vi "rt nominal connect.vi"(8 "error in":errorcluster, 11 "stream configuration":T5={"stream name"="", "Base URL"="https://api.gov.nominal.io/api/", "api key"="", "identifier selection"=enum."Asset Identifier and Dataset Name", "asset ID"="", "dataset name"="", "dataset ID"="", "associated channels"=[], "fallback avro path"=path "", "time source"=enum."to timestamp", "buffer size"=0}) -> (0 "error out":errorcluster, 2 "channel buffer":T1, 3 "nominal state":T3)   [LabVIEW 2026, in "Nominal Core Streaming Engine.lvlib"]
uses:
  Nominal Core Streaming Engine.lvlib
  Shared/compiled stream data.ctl
  Shared/stream configuration mode.ctl
  Shared/time convert type.ctl
  nominal runtime state.ctl
  rt full channel buffer.ctl
  rt per channel buffer.ctl
  <vilib>/Utility/sysdir.llb/System Directory Type.ctl
  Shared/Nominal Core Streaming Shared.lvlib
  lib_nominal-streaming-lv_64.dll
  libnominalClient_64.dll
panel:
  out "out_stream_handle":u64
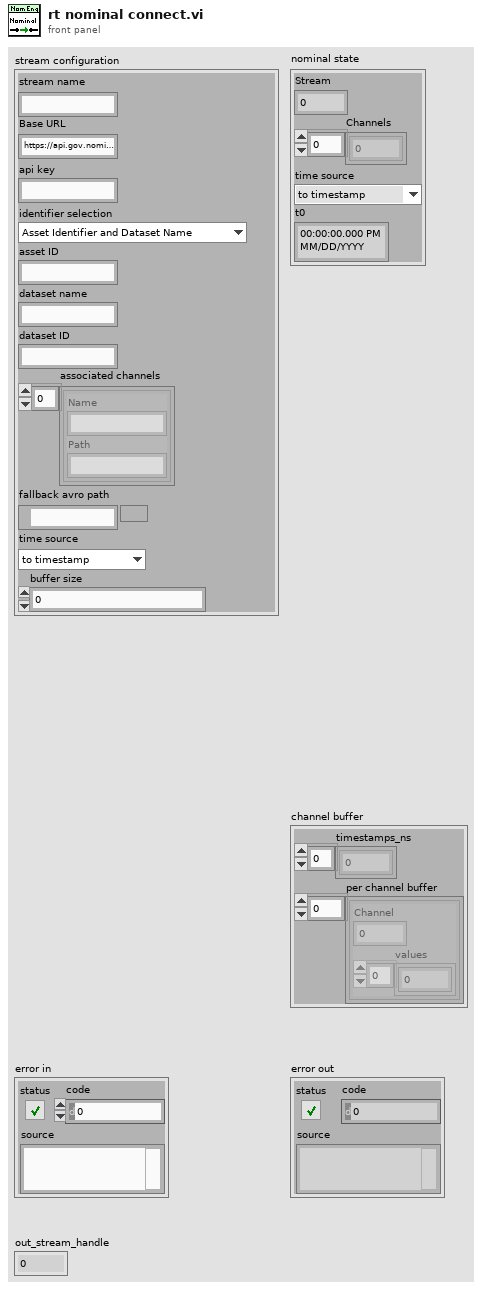
[diagram p1: front panel]
types:
  T1 = typedef "Nominal Core Streaming Engine.lvlib/rt full channel buffer.ctl" = cluster{"timestamps_ns":i64[], "per channel buffer":T2[]}
  T2 = typedef "Nominal Core Streaming Engine.lvlib/rt per channel buffer.ctl" = cluster{"Channel":u64, "values":dbl[]}
  T3 = typedef "Nominal Core Streaming Engine.lvlib/nominal runtime state.ctl" = cluster{"Stream":u64, "Channels":u64[], "time source":T4, "t0":timestamp}
  T4 = typedef "Nominal Core Streaming Shared.lvlib/time convert type.ctl" = enum16{"to timestamp", "relative seconds"}
  T5 = typedef "Nominal Core Streaming Shared.lvlib/compiled stream data.ctl" = cluster{"stream name":string, "Base URL":string, "api key":string, "identifier selection":T6, "asset ID":string, "dataset name":string, "dataset ID":string, "associated channels":cluster{"Name":string, "Path":string}[], "fallback avro path":path, "time source":T4, "buffer size":u32}
  T6 = typedef "Nominal Core Streaming Shared.lvlib/stream configuration mode.ctl" = enum16{"Asset Identifier and Dataset Name", "Dataset Identifier"}
  T7 = typedef "System Directory Type.ctl" = i32
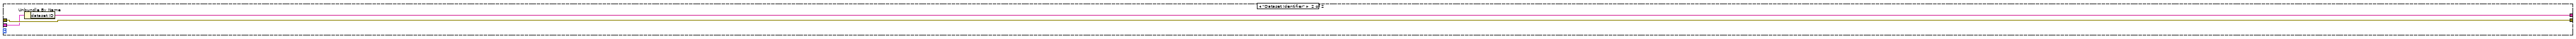
[diagram p4: hidden frame]
diagram:
  n1 = Unbundle By Name("stream configuration") -> ("associated channels"=w15:cluster{"Name":string, "Path":string}[])
  n2 = Unbundle By Name("stream configuration") -> ("identifier selection"=w21:T6)
  n3 = Unbundle By Name("stream configuration") -> ("fallback avro path"=w19:path)
  n4 = Unbundle By Name("stream configuration") -> ("time source"=w9:T4)
  n5 = Unbundle By Name("stream configuration") -> ("buffer size"=w4:u32)
  n6 = case shown="\"Asset Identifier and Dataset Name\"" w21 {
    tunnel: "error in" -> [w29 w164]
    tunnel: [w25 w164] -> w2
    tunnel: "stream configuration" -> [w23 w163]
    tunnel: [w28 w162] -> w1
    frame "Asset Identifier and Dataset Name" {
      n7 = flat-sequence {
        tunnel: [w53] -> w36
        tunnel: [w52] -> w35
        tunnel: w29 -> [w51]
        tunnel: [w49] -> w26
        tunnel: [w48] -> w24
        tunnel: w23 -> [w38]
        frame #0 {
          n8 = Unbundle By Name(w38) -> ("api key"=w39:string, "Base URL"=w40:string)
          n9 = Unbundle By Name(w38) -> ("asset ID"=w37:string)
          n10 = dll-call lib="C:/sw/ni-veristand-custom-device-nominal-core/source/libnominalClient_*.*" fn="nominal_client_new"(error in=w51, "token"=w39, "workspace_rid"="", "base_url"=w40) -> (error out=w42:errorcluster, "return type"=w41:i32, "out_client"=w48:i32)  [unwired: 6 in, 1 out]
          n11 = call "extracted dll error handler.vi"("error in (no error)"=w42, "error code"=w41) -> ("error out"=w50:errorcluster)  [unwired: 9 in]
          n12 = dll-call lib="C:/sw/ni-veristand-custom-device-nominal-core/source/libnominalClient_*.*" fn="nominal_asset_get"(error in=w50, "client"=w48, "rid"=w37) -> (error out=w45:errorcluster, "return type"=w44:i32, "out_asset"=w49:i32)  [unwired: 5 in, 1 out]
          n13 = call "extracted dll error handler.vi"("error in (no error)"=w45, "error code"=w44) -> ("error out"=w54:errorcluster)  [unwired: 9 in]
          n14 = dll-call lib="C:/sw/ni-veristand-custom-device-nominal-core/source/libnominalClient_*.*" fn="nominal_asset_data_source_count"(error in=w54, "asset"=w49) -> (error out=w47:errorcluster, "return type"=w46:i32, "out_count"=w52:u32)  [unwired: 4 in, 1 out]
          n15 = call "extracted dll error handler.vi"("error in (no error)"=w47, "error code"=w46) -> ("error out"=w53:errorcluster)  [unwired: 9 in]
        }
      }
      n16 = for {
        N: w35 -> [_]
        shift-right: [w93] -> w31
        shift-left: w36 -> [w95]
        tunnel: w26 -> [w91]
        tunnel: [w89] -> w30
        tunnel: [w88] -> w34
        tunnel: w24 -> [w87]
        tunnel: w23 -> [w86]
        i -> [w90]
        stop <- w88 stop-if-true
        n17 = flat-sequence {
          tunnel: w95 -> [w102]
          tunnel: [w101] -> w94
          tunnel: [w100] -> w92
          tunnel: w91 -> [w99]
          tunnel: w90 -> [w98]
          frame #0 {
            # "NominalDataSourceType_Dataset = 0,\n  NominalDataSourceType_Video = 1,\n  NominalDataSourceType_Connection = 2,"
            n18 = dll-call lib="C:/sw/ni-veristand-custom-device-nominal-core/source/libnominalClient_*.*" fn="nominal_asset_data_source_type_at"(error in=w102, "asset"=w99, "index"=w98) -> (error out=w97:errorcluster, "return type"=w96:i32, "out_type"=w101:i32)  [unwired: 5 in, 1 out]
            n19 = call "extracted dll error handler.vi"("error in (no error)"=w97, "error code"=w96) -> ("error out"=w100:errorcluster)  [unwired: 9 in]
          }
        }
        n20 = case shown="0" w94 {
          tunnel: [w105 w161] -> w93
          tunnel: w92 -> [w119 w161]
          tunnel: w91 -> [w118 _]
          tunnel: w90 -> [w114 _]
          tunnel: [w110 _] -> w89
          tunnel: [w107 _] -> w88
          tunnel: w87 -> [w111 _]
          tunnel: w86 -> [w104 _]
          frame 0 {
            # "I personally find scope name vs dataset name to be extremely confusing, so I'm checking both"
            n21 = stacked-sequence {
              tunnel: [w132] -> w117
              tunnel: [w128] -> w116
              tunnel: [w125] -> _
              tunnel: [w129] -> _
              tunnel: w119 -> [w130]
              tunnel: w114 -> [w127]
              tunnel: w118 -> [w126]
              frame #0 {
                n22 = call "extracted create string buffer.vi"("Buffer Size (1024)"=2048 ("dimension size")) -> ("dub Buffer Size"=w123:i32, "String Buffer"=w122:string)  [unwired: 8 in, 1 out]
                n23 = dll-call lib="C:/sw/ni-veristand-custom-device-nominal-core/source/libnominalClient_*.*" fn="nominal_asset_data_source_name_at"(error in=w130, "asset"=w126, "index"=w127, "buf"=w122, "cap"=w123) -> (error out=w131:errorcluster, "return type"=w125:i32, "buf"=w128:string, "out_needed"=w129:u32)  [unwired: 6 in, 1 out]
                n24 = call "extracted dll error handler.vi"("error in (no error)"=w131, "error code"=w125) -> ("error out"=w132:errorcluster)  [unwired: 9 in]
              }
            }
            n25 = Unbundle By Name(w104) -> ("dataset name"=w103:string)
            n26 = Equal?(x=w103, y=w116) -> (x = y?=w115:bool)
            n27 = stacked-sequence {
              tunnel: [w143] -> w112
              tunnel: [w139] -> w110
              tunnel: [w136] -> _
              tunnel: [w140] -> _
              tunnel: w117 -> [w141]
              tunnel: w114 -> [w138]
              tunnel: w118 -> [w137]
              frame #0 {
                n28 = call "extracted create string buffer.vi"("Buffer Size (1024)"=2048 ("dimension size")) -> ("dub Buffer Size"=w134:i32, "String Buffer"=w133:string)  [unwired: 8 in, 1 out]
                n29 = dll-call lib="C:/sw/ni-veristand-custom-device-nominal-core/source/libnominalClient_*.*" fn="nominal_asset_data_source_rid_at"(error in=w141, "asset"=w137, "index"=w138, "buf"=w133, "cap"=w134) -> (error out=w142:errorcluster, "return type"=w136:i32, "buf"=w139:string, "out_needed"=w140:u32)  [unwired: 6 in, 1 out]
                n30 = call "extracted dll error handler.vi"("error in (no error)"=w142, "error code"=w136) -> ("error out"=w143:errorcluster)  [unwired: 9 in]
              }
            }
            n31 = stacked-sequence {
              tunnel: [w160] -> w109
              tunnel: [w157] -> w113
              tunnel: [w154] -> _
              tunnel: w112 -> [w158]
              tunnel: w110 -> [w156]
              tunnel: w111 -> [w155]
              frame #0 {
                n32 = dll-call lib="C:/sw/ni-veristand-custom-device-nominal-core/source/libnominalClient_*.*" fn="nominal_dataset_get"(error in=w158, "client"=w155, "rid"=w156) -> (error out=w159:errorcluster, "return type"=w154:i32, "out_dataset"=w157:i32)  [unwired: 5 in, 1 out]
                n33 = call "extracted dll error handler.vi"("error in (no error)"=w159, "error code"=w154) -> ("error out"=w160:errorcluster)  [unwired: 9 in]
              }
            }
            n34 = stacked-sequence {
              tunnel: [w153] -> w105
              tunnel: [w149] -> w108
              tunnel: [w147] -> _
              tunnel: [w150] -> _
              tunnel: w109 -> [w151]
              tunnel: w113 -> [w148]
              frame #0 {
                n35 = call "extracted create string buffer.vi"("Buffer Size (1024)"=2048 ("dimension size")) -> ("dub Buffer Size"=w145:i32, "String Buffer"=w144:string)  [unwired: 8 in, 1 out]
                n36 = dll-call lib="C:/sw/ni-veristand-custom-device-nominal-core/source/libnominalClient_*.*" fn="nominal_dataset_name"(error in=w151, "dataset"=w148, "buf"=w144, "cap"=w145) -> (error out=w152:errorcluster, "return type"=w147:i32, "buf"=w149:string, "out_needed"=w150:u32)  [unwired: 5 in, 1 out]
                n37 = call "extracted dll error handler.vi"("error in (no error)"=w152, "error code"=w147) -> ("error out"=w153:errorcluster)  [unwired: 9 in]
              }
            }
            n38 = Equal?(x=w103, y=w108) -> (x = y?=w106:bool)
            n39 = flat-sequence {
              tunnel: w113 -> [w121]
              tunnel: w105 -> [_]
              tunnel: [w120] -> _
              frame #0 {
                n40 = dll-call lib="C:/sw/ni-veristand-custom-device-nominal-core/source/libnominalClient_*.*" fn="nominal_dataset_free"("dataset"=w121) -> (error out=w120:errorcluster)  [unwired: 5 in, 1 out]
              }
            }
            n41 = Or(x=w106, y=w115) -> (x .or. y?=w107:bool)
          }
          frame Default {
          }
        }
      }
      n42 = Empty String/Path?(string/path=w30) -> (empty?=w33:bool)
      n43 = Compound Arithmetic op=AND(invert w33, w34) -> (w32:bool)
      n44 = case shown="False" w32 {
        tunnel: w31 -> [w81 w85]
        tunnel: w24 -> [w71 _]
        tunnel: w30 -> [_ w84]
        tunnel: [w73 w85] -> w25
        tunnel: [w66 w84] -> w28
        tunnel: w23 -> [w69 _]
        frame False {
          # "not found on asset, create and attach"
          n45 = Unbundle By Name(w69) -> ("dataset name"=w67:string, "stream name"=w68:string)
          n46 = dll-call lib="C:/sw/ni-veristand-custom-device-nominal-core/source/libnominalClient_*.*" fn="nominal_dataset_create"(error in=w81, "client"=w71, "name"=w67, "description"=w68) -> (error out=w65:errorcluster, "return type"=w64:i32, "out_dataset"=w72:i32)  [unwired: 6 in, 1 out]
          n47 = Unbundle By Name(w69) -> ("asset ID"=w70:string, "dataset name"=w59:string)
          n48 = call "extracted dll error handler.vi"("error in (no error)"=w65, "error code"=w64) -> ("error out"=w75:errorcluster)  [unwired: 9 in]
          n49 = call "extracted create string buffer.vi"("error in"=w75, "Buffer Size (1024)"=2048) -> ("error out"=w79:errorcluster, "dub Buffer Size"=w77:i32, "String Buffer"=w78:string)  [unwired: 7 in]
          n50 = dll-call lib="C:/sw/ni-veristand-custom-device-nominal-core/source/libnominalClient_*.*" fn="nominal_dataset_rid"(error in=w79, "dataset"=w72, "buf"=w78, "cap"=w77, "out_needed"=u32 0) -> (error out=w61:errorcluster, "return type"=w60:i32, "buf"=w66:string)  [unwired: 5 in, 1 out]
          n51 = call "extracted dll error handler.vi"("error in (no error)"=w61, "error code"=w60) -> ("error out"=w74:errorcluster)  [unwired: 9 in]
          n52 = dll-call lib="C:/sw/ni-veristand-custom-device-nominal-core/source/libnominalClient_*.*" fn="nominal_asset_add_dataset"(error in=w74, "client"=w71, "rid"=w70, "scope_name"=w59, "dataset_rid"=w66) -> (error out=w63:errorcluster, "return type"=w62:i32, "out_asset"=w80:i32)  [unwired: 7 in, 1 out]
          n53 = flat-sequence {
            tunnel: w80 -> [w82]
            tunnel: w72 -> [w83]
            frame #0 {
              # "int32_t nominal_asset_free(int32_t asset);"
              n54 = dll-call lib="C:/sw/ni-veristand-custom-device-nominal-core/source/libnominalClient_*.*" fn="nominal_asset_free"("asset"=w82) -> ()  [unwired: 5 in, 2 out]
            }
            frame #1 {
              # "int32_t nominal_dataset_free(int32_t dataset);"
              n55 = dll-call lib="C:/sw/ni-veristand-custom-device-nominal-core/source/libnominalClient_*.*" fn="nominal_dataset_free"("dataset"=w83) -> ()  [unwired: 5 in, 2 out]
            }
          }
          n56 = call "extracted dll error handler.vi"("error in (no error)"=w63, "error code"=w62) -> ("error out"=w73:errorcluster)  [unwired: 9 in]
        }
        frame True {
          # "exists and is part of asset"
        }
      }
      n57 = flat-sequence {
        tunnel: w24 -> [w56]
        tunnel: [w56] -> w27
        tunnel: w26 -> [w55]
        tunnel: w25 -> [_]
        tunnel: w27 -> [w57]
        frame #0 {
          # "int32_t nominal_asset_free(int32_t asset);"
          n58 = dll-call lib="C:/sw/ni-veristand-custom-device-nominal-core/source/libnominalClient_*.*" fn="nominal_asset_free"("asset"=w55) -> ()  [unwired: 5 in, 2 out]
        }
        frame #1 {
          # "int32_t nominal_client_free(int32_t client);"
          n59 = dll-call lib="C:/sw/ni-veristand-custom-device-nominal-core/source/libnominalClient_*.*" fn="nominal_client_free"("client"=w57) -> ()  [unwired: 5 in, 2 out]
        }
      }
    }
    frame "Dataset Identifier" {
      n60 = Unbundle By Name(w163) -> ("dataset ID"=w162:string)
    }
  }
  n61 = call "reprocess channel names for duplicates.vi"("channels in"=w15) -> ("processed channels"=w14:cluster{"Name":string, "Path":string}[])  [unwired: 10 in]
  n62 = stacked-sequence {
    tunnel: [w177] -> w20
    tunnel: w19 -> [w188]
    tunnel: w2 -> [w191]
    tunnel: [w176] -> w7
    tunnel: "stream configuration" -> [w174]
    tunnel: w1 -> [w165]
    frame #0 {
      w183 = T7 2 items=["User Home"=0, "User Desktop"=1, "User Documents"=2, "User Application Data"=3, "User Preferences"=4, "User Temporary"=5, "Public Documents"=6, "Public Application Data"=7, "Public Preferences"=8, "Public Cache"=13, "System Core Libraries"=9, "System Installed Libraries"=10, "Application Files"=11, "Boot Volume Root"=12] ("system directory type")
      # "streaming setup"
      n63 = Unbundle By Name(w174) -> ("api key"=w175:string)
      n64 = call <vilib>:"Get System Directory.vi"("system directory type"=w183) -> ("system directory"=w182:path)  [unwired: 10 in]
      n65 = Get Date/Time In Seconds() -> (seconds since 1Jan1904=w180:timestamp)
      n66 = Build Path(base path=w182, name or relative path=path "nominal_fallback_files") -> (appended path=w184:path)
      n67 = Format Into String(format string="%<%Y-%m-%d_%H-%M_fallback-file.avro>T", error in=w191, w180) -> (resulting string=w181:string, error out=w186:errorcluster)  [unwired: 1 in]
      n68 = call <vilib>:"Is Path and Not Empty.vi"("path"=w188) -> ("Is Path and Not Empty?"=w187:bool)  [unwired: 4 in]
      n69 = call <vilib>:"Create Directory Recursive.vi"("error in (no error)"=w186, "directory"=w184) -> ("directory copy"=w185:path)  [unwired: 3 in, 2 out]
      n70 = Build Path(base path=w185, name or relative path=w181) -> (appended path=w189:path)
      n71 = Select(t=w188, s=w187, f=w189) -> (s? t:f=w190:path)
      n72 = Path To String(path=w190) -> (string=w172:string)
      n73 = dll-call lib="C:/sw/ni-veristand-custom-device-nominal-core/source/lib_nominal-streaming-lv_*.*" fn="nominal_init"(error in=w191, "token"=w175, "dataset_rid"=w165, "fallback_file_path"=w172, "out_stream_handle"=u64 0) -> (error out=w173:errorcluster, "out_stream_handle"=w176:u64)  [unwired: 6 in, 1 out]
      n74 = call "extracted create string buffer.vi"() -> ("dub Buffer Size"=w166:i32, "String Buffer"=w167:string)  [unwired: 9 in, 1 out]
      n75 = dll-call lib="C:/sw/ni-veristand-custom-device-nominal-core/source/lib_nominal-streaming-lv_*.*" fn="nominal_get_last_error"(error in=w173, "buffer"=w167, "buffer_size"=w166) -> (error out=w168:errorcluster, "return type"=w170:i32, "buffer"=w169:string)  [unwired: 3 in, 1 out]
      n76 = case shown="Default" w170 {
        tunnel: w168 -> [w192 w197]
        tunnel: [w192 w196] -> w177
        tunnel: w169 -> [_ w195]
        frame -1 {
        }
        frame Default {
          n77 = call <vilib>:"Error Cluster From Error Code.vi"("show call chain? (False)"=TRUE, "error in (no error)"=w197, "error message (\"\")"=w195, "error code (0)"=5001) -> ("error out"=w196:errorcluster)  [unwired: 5 in]
        }
      }
    }
  }
  "out_stream_handle" <- w7
  n78 = for {
    shift-right: [w210] -> w16
    shift-left: w20 -> [w211]
    tunnel: w14 -> [w208] mode=indexing
    tunnel: [w203] -> w11 mode=indexing
    tunnel: w4 -> [w200]
    tunnel: [w198] -> w8 mode=indexing
    tunnel: w7 -> [w199]
    n79 = Unbundle(w208) -> ("Name"=w205:string, "Path"=w207:string)
    n80 = node("nivs_path" ("key"), w207) -> (w209:map{string, string})
    n81 = stacked-sequence {
      tunnel: [w225] -> w210
      tunnel: w211 -> [w219]
      tunnel: w209 -> [w221]
      tunnel: w205 -> [w227]
      tunnel: [w218] -> w198
      tunnel: w199 -> [w217]
      frame #0 {
        n82 = for {
          tunnel: w221 -> [w238] mode=indexing
          tunnel: [w234] -> w222 mode=indexing
          n83 = Unbundle By Name(w238) -> ("key"=w237:string, "Path"=w236:string)
          n84 = Concatenate Strings(w237, "=" ("string"), w236) -> (w234:string)
        }
        n85 = call <vilib>:"1D String Array to Delimited String.vi"("delimiter"=",", "string array"=w222) -> ("delimited string"=w226:string)  [unwired: 9 in]
        n86 = dll-call lib="C:/sw/ni-veristand-custom-device-nominal-core/source/lib_nominal-streaming-lv_*.*" fn="nominal_create_channel"(error in=w219, "stream_handle"=w217, "channel_name"=w227, "tags_csv"=w226, "out_writer_handle"=u64 0) -> (error out=w224:errorcluster, "out_writer_handle"=w218:u64)  [unwired: 6 in, 1 out]
        n87 = call "extracted create string buffer.vi"() -> ("dub Buffer Size"=w212:i32, "String Buffer"=w213:string)  [unwired: 9 in, 1 out]
        n88 = dll-call lib="C:/sw/ni-veristand-custom-device-nominal-core/source/lib_nominal-streaming-lv_*.*" fn="nominal_get_last_error"(error in=w224, "buffer"=w213, "buffer_size"=w212) -> (error out=w214:errorcluster, "return type"=w216:i32, "buffer"=w215:string)  [unwired: 3 in, 1 out]
        n89 = case shown="Default" w216 {
          tunnel: w214 -> [w228 w233]
          tunnel: [w228 w232] -> w225
          tunnel: w215 -> [_ w231]
          frame -1 {
          }
          frame Default {
            n90 = call <vilib>:"Error Cluster From Error Code.vi"("show call chain? (False)"=TRUE, "error in (no error)"=w233, "error message (\"\")"=w231, "error code (0)"=5002) -> ("error out"=w232:errorcluster)  [unwired: 5 in]
          }
        }
      }
    }
    n91 = Initialize Array(0.0 ("Numeric"), w200) -> (w201:dbl[])
    n92 = Bundle By Name(cluster=T2 {"Channel"=0, "values"=[]} ("channel buffer"), "Channel"=w198, "values"=w201) -> (w203:T2)
  }
  "error out" <- w16
  n93 = Get Date/Time In Seconds() -> (seconds since 1Jan1904=w5:timestamp)
  n94 = call "extracted timestamp to ns.vi"("Time Stamp"=w5) -> ("nominal core ns"=w6:i64)  [unwired: 10 in]
  n95 = Initialize Array(w6, w4) -> (w12:i64[])
  n96 = Bundle By Name(cluster=T1 {"timestamps_ns"=[], "per channel buffer"=[]} ("channel buffer"), "timestamps_ns"=w12, "per channel buffer"=w11) -> (→"channel buffer":T1)
  n97 = Bundle By Name(cluster=T3 {"Stream"=0, "Channels"=[], "time source"=enum."to timestamp", "t0"=timestamp(0 s since 1904-01-01)} ("nominal state"), "Stream"=w7, "Channels"=w8, "time source"=w9, "t0"=w5) -> (→"nominal state":T3)
